vi "Autonomous Independent.vi"() -> ()   [LabVIEW 2013]
doc: "This VI is called when autonomous begins, and will automatically be terminated when autonomous ends. You can carry out timed or sensor driven robot movement independently without needing to return to the caller."
uses:
  Robot Global Data.vi
panel:
  in  "HighGear?":bool
  in  "error":errorcluster
  out "Hot?":bool
  in  "Drive?":bool
  in  "DesiredMotorInput":dbl=0.4
  in  "% Cutoff":dbl=0.5
  in  "Num samples":i32=5
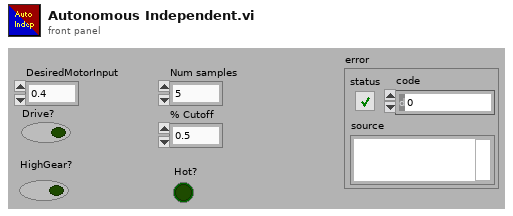
[diagram p1: front panel]
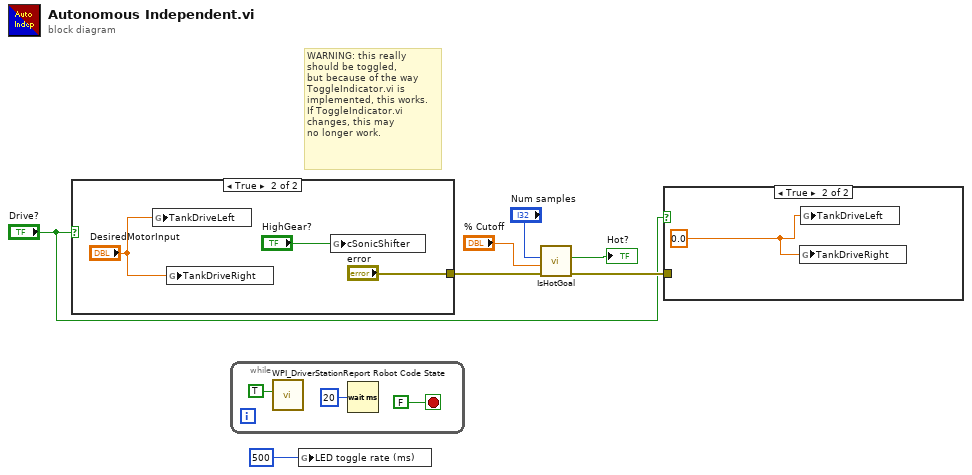
[diagram p0: block diagram]
diagram:
  # "WARNING: this really \nshould be toggled,\nbut because of the way\nToggleIndicator.vi is \nimplemented, this works.\nIf ToggleIndicator.vi \nchanges, this may\nno longer work."
  n1 = case shown="True" "Drive?" {
    tunnel: [_ "error"] -> w4
    frame False {
    }
    frame True {
      n2 = global write "Robot Global Data.vi" "TankDriveLeft"("DesiredMotorInput") -> ()
      n3 = global write "Robot Global Data.vi" "TankDriveRight"("DesiredMotorInput") -> ()
      n4 = global write "Robot Global Data.vi" "cSonicShifter"("HighGear?") -> ()
    }
  }
  n5 = while {
    stop <- FALSE stop-if-true
    n6 = call <vilib>:"WPI_DriverStationReport Robot Code State.vi"("Autonomous"=TRUE) -> ()  [unwired: 10 in, 1 out]
    n7 = Wait (ms)(milliseconds to wait=u32 20) -> ()  [unwired: 1 out]
  }
  n8 = global write "Robot Global Data.vi" "LED toggle rate (ms)"(u32 500 ("LED ms toggle rate")) -> ()
  n9 = call "IsHotGoal.vi"("error in"=w4, "% Cutoff"="% Cutoff", "Num samples"="Num samples") -> ("error out"=w2:errorcluster, "Hot/Not"=→"Hot?":bool)  [unwired: 7 in]
  n10 = case shown="True" "Drive?" {
    tunnel: w2 -> [_ _]
    frame False {
    }
    frame True {
      w14 = 0.0 ("RightDesired")
      n11 = global write "Robot Global Data.vi" "TankDriveRight"(w14) -> ()
      n12 = global write "Robot Global Data.vi" "TankDriveLeft"(w14) -> ()
    }
  }
